vi "Laser Off (SubVI).vi"(8 "error in (no error)":errorcluster) -> (0 "error out":errorcluster, 2 "ASG Connection on":bool, 3 "Laser On":bool)   [LabVIEW 2020]
uses:
  Labview Library/Libraries/ASG8100CY/ASG8X00_x64.dll
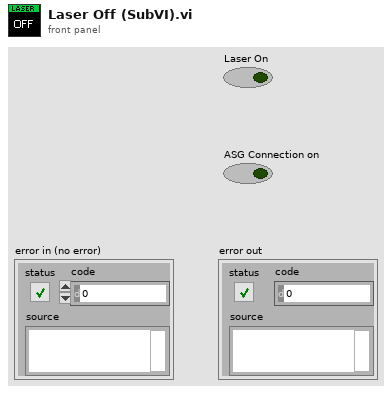
[diagram p1: front panel]
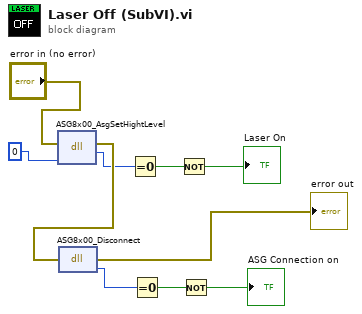
[diagram p0: block diagram]
diagram:
  n1 = dll-call lib="F:/Labview Library/Libraries/ASG8100CY/ASG8X00_x64.dll" fn="ASG8x00_AsgSetHightLevel"(error in="error in (no error)", "参数1"=0) -> (error out=w7:errorcluster, "返回类型"=w2:i32)  [unwired: 3 in, 1 out]
  n2 = dll-call lib="F:/Labview Library/Libraries/ASG8100CY/ASG8X00_x64.dll" fn="ASG8x00_Disconnect"(error in=w7) -> (error out=→"error out":errorcluster, "return type"=w9:i32)  [unwired: 2 in, 1 out]
  n3 = Equal To 0?(x=w2) -> (x = 0?=w3:bool)
  n4 = Equal To 0?(x=w9) -> (x = 0?=w5:bool)
  n5 = Not(x=w3) -> (.not. x?=→"Laser On":bool)
  n6 = Not(x=w5) -> (.not. x?=→"ASG Connection on":bool)
